vi "Configuration.vi"() -> ()   [LabVIEW 2017]
doc: "Demonstrates how to:\n- Discover SLSC devices\n- Reset SLSC devices\n- Rename SLSC devices\n- Add/remove SLSC chassis to/from the SLSC configuration file\n- Log in/out of an SLSC chassis, caching/deleting its login credentials\n- Update the firmware for an SLSC chassis\n- Open the web configuration page for an SLSC chassis"
uses:
  ConfigurationStates.ctl
  <vilib>/SLSC/Initialize Session without Resources.vi
  <vilib>/SLSC/Initialize Session with Devices.vi
  <vilib>/SLSC/Close Session.vi
  <vilib>/Platform/browser.llb/Open URL in Default Browser (string).vi
  <vilib>/SLSC/SLSC.lvlib
  <resource>/objmgr/slsc.rc
panel:
  in  "web config":bool
  in  "update firmware":bool
  out "device properties":string[][](table)
  in  "refresh":bool
  in  "logout":bool
  in  "login":bool
  in  "rename":bool
  in  "reset":bool
  in  "stop":bool
  in  "remove":bool
  in  "add":bool
  in  "devices":string(tree)="jasonSlsc-5"
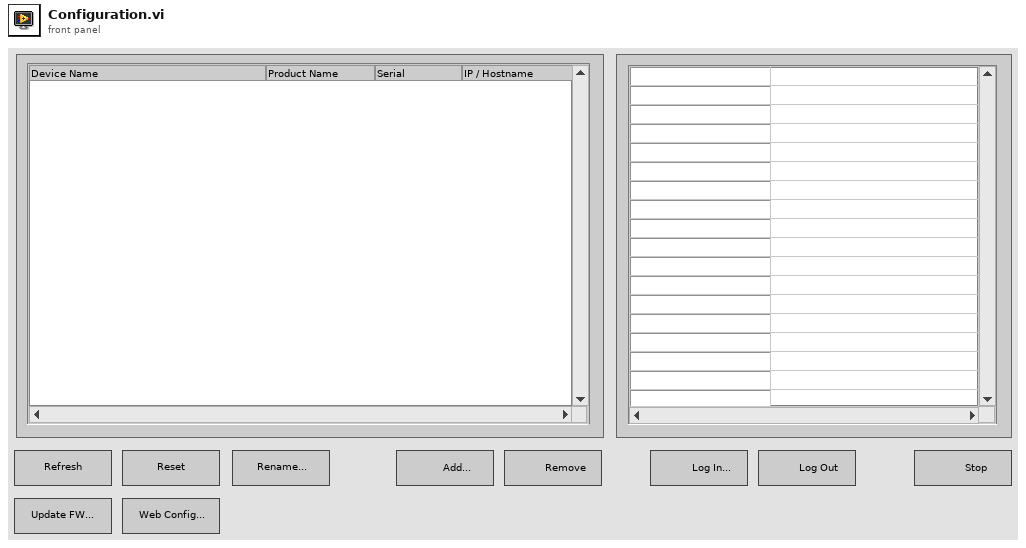
[diagram p1: front panel]
types:
  T1 = typedef "ConfigurationStates.ctl" = enum16{"Add", "Remove", "Rename", "Reset", "Login", "Logout", "Stop", "Refresh", "Update Firmware", "Web Config"}
  T2 = enum8{"Enabled", "Disabled", "Disabled and Grayed Out"}
  T3 = cluster{"hostname":string, "username":string, "password":string}
  T4 = cluster{"username":string, "password":string, "save credentials to disk":bool}
  T5 = cluster{"firmware path":path, "username":string, "password":string}
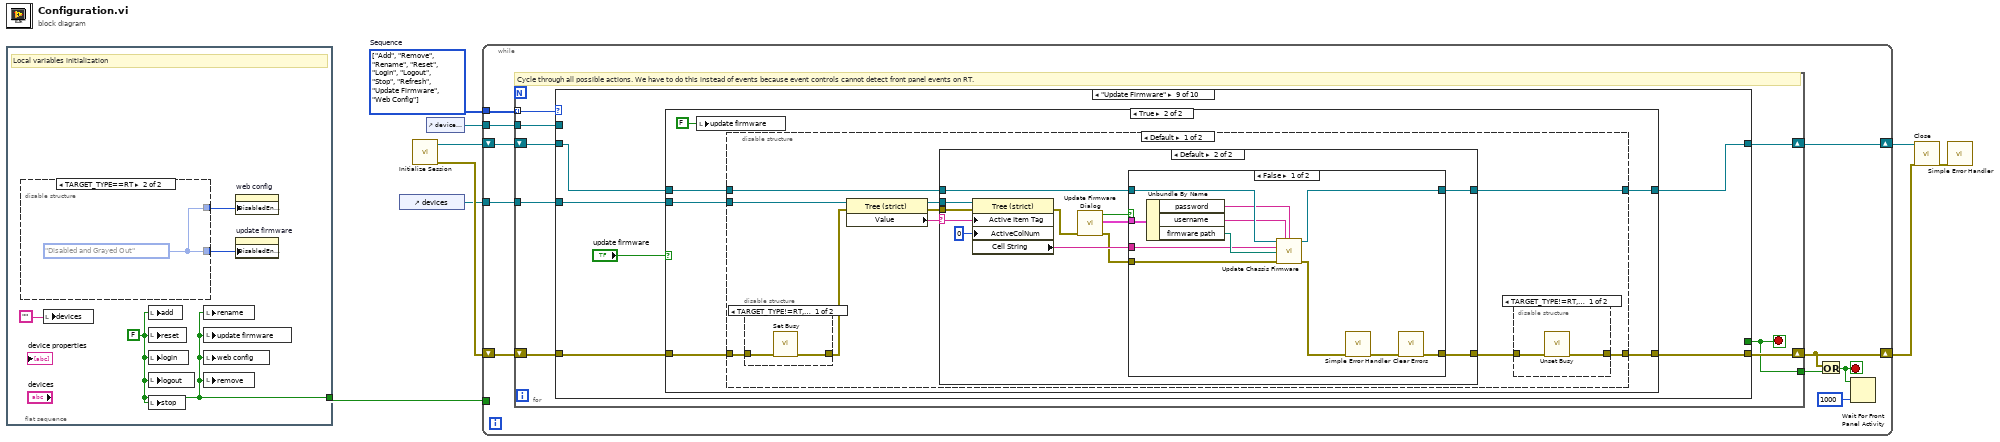
[diagram p0: block diagram]
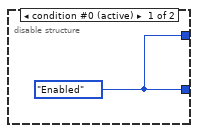
[diagram p2: hidden frame]
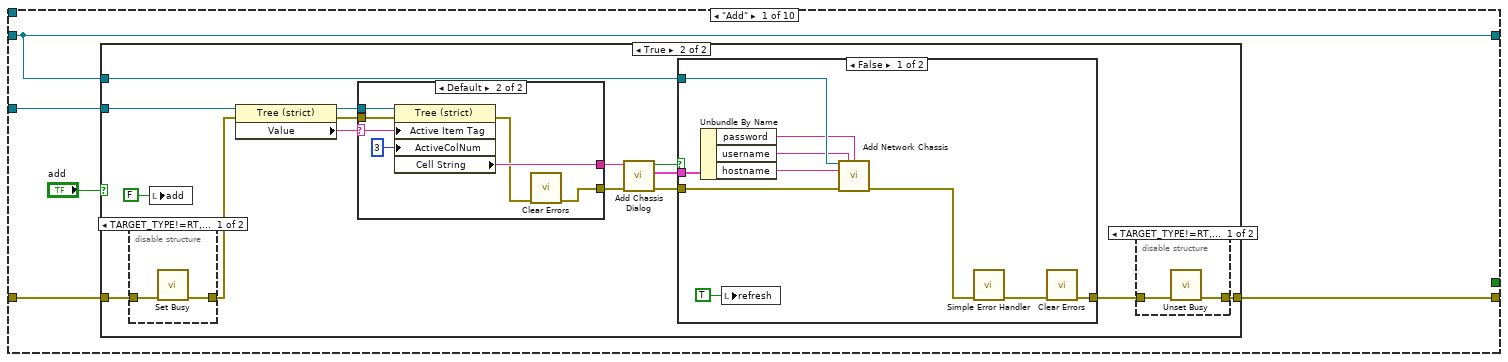
[diagram p3: hidden frame]
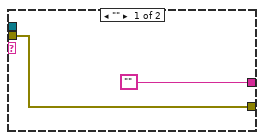
[diagram p5: hidden frame]
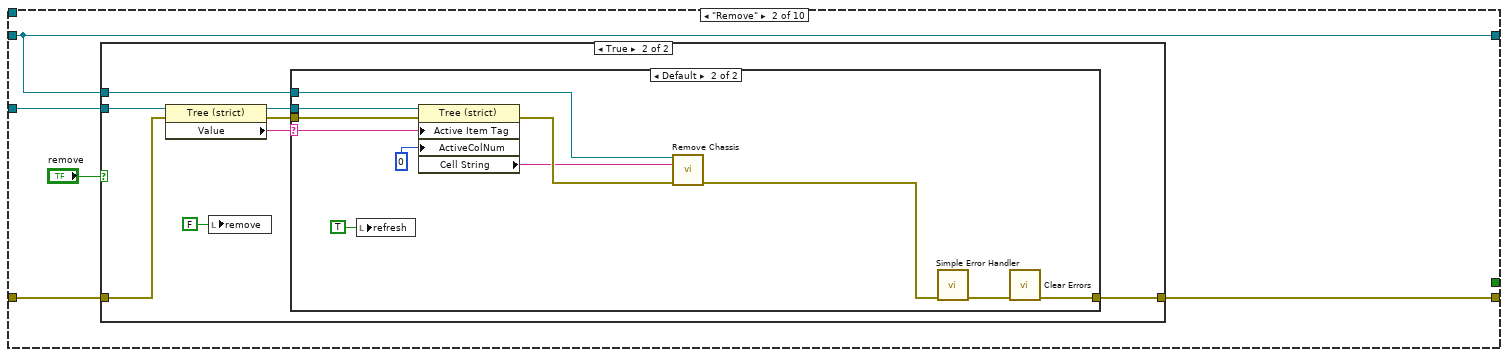
[diagram p9: hidden frame]
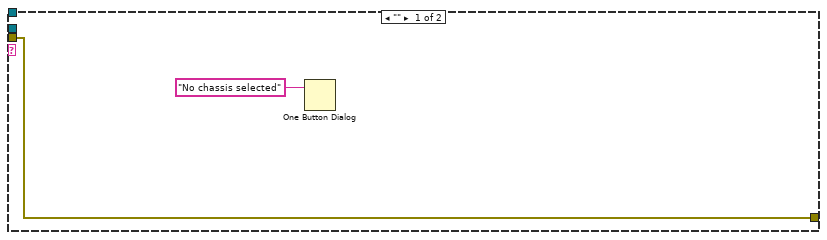
[diagram p11: hidden frame]
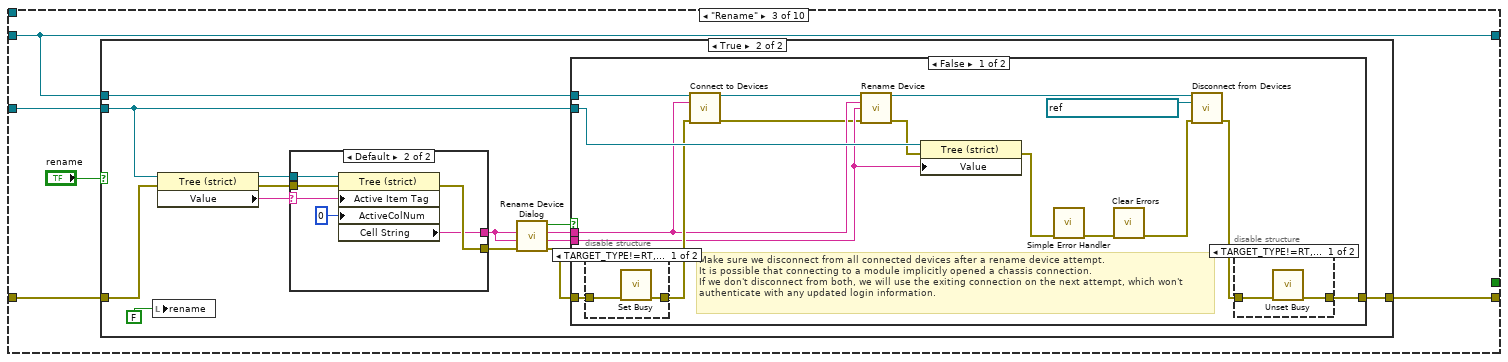
[diagram p12: hidden frame]
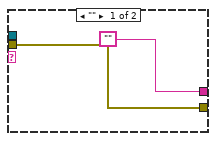
[diagram p14: hidden frame]
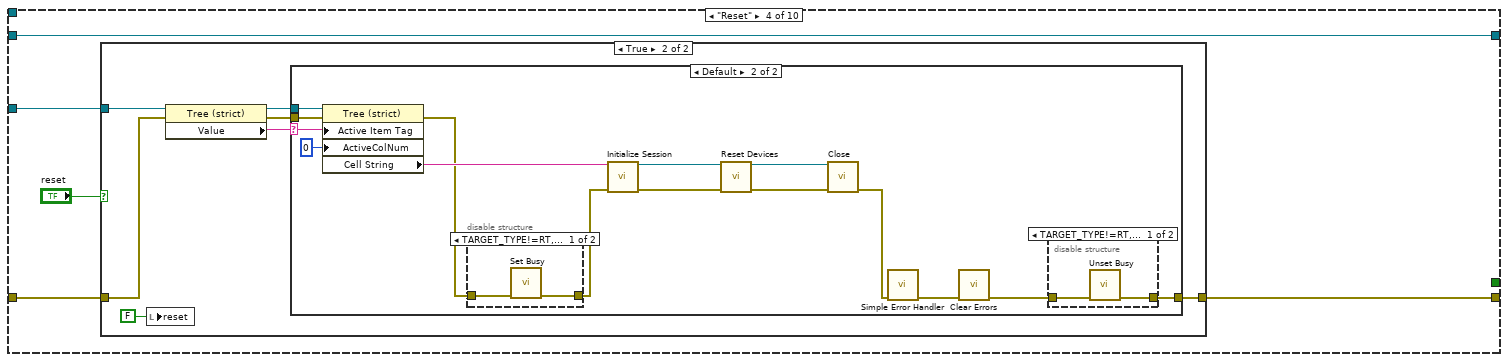
[diagram p18: hidden frame]
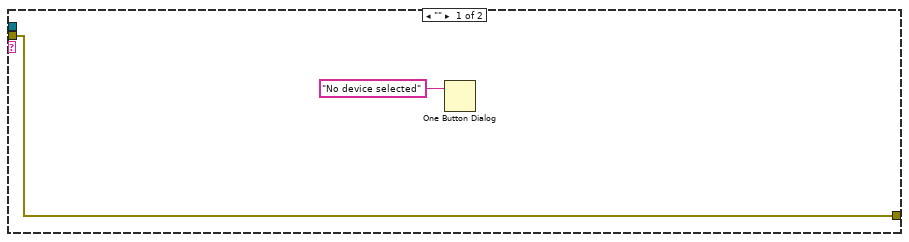
[diagram p20: hidden frame]
diagram:
  w4 = T1[] [enum."Add", enum."Remove", enum."Rename", enum."Reset", enum."Login", enum."Logout", enum."Stop", enum."Refresh", enum."Update Firmware", enum."Web Config"] items=["Add", "Remove", "Rename", "Reset", "Login", "Logout", "Stop", "Refresh", "Update Firmware", "Web Config"]  # Sequence
  n1 = flat-sequence {
    tunnel: [w13] -> w3
    frame #0 {
      w13 = FALSE
      # "Local variables initialization"
      n2 = disable-structure shown="TARGET_TYPE==RT" {
        disable-tunnel: [w14 w15] -> w12
        disable-tunnel: [w14 w15] -> w10
        frame condition #0 (active) {
          w14 = T2."Enabled" ("Disabled")
        }
        frame condition #1 {
          w15 = T2."Disabled and Grayed Out" ("Disabled")
        }
      }
      n3 = local write "devices"("") -> ()
      n4 = local write "add"(w13) -> ()
      n5 = local write "reset"(w13) -> ()
      n6 = local write "login"(w13) -> ()
      n7 = local write "logout"(w13) -> ()
      n8 = local write "stop"(w13) -> ()
      n9 = local write "rename"(w13) -> ()
      n10 = local write "update firmware"(w13) -> ()
      n11 = local write "web config"(w13) -> ()
      n12 = local write "remove"(w13) -> ()
      n13 = property on="web config" class="Bool (strict)"("DisabledEnum"=w10) -> ()  [unwired: 2 in, 2 out]
      n14 = property on="update firmware" class="Bool (strict)"("DisabledEnum"=w12) -> ()  [unwired: 2 in, 2 out]
    }
  }
  n15 = control-ref of="devices"() -> (w5:refnum<vi>)
  n16 = call-poly <vilib>:"Initialize Session.vi"() -> ("session out"=w6:refnum<k21>, "error out"=w9:errorcluster)  [unwired: 14 in]
  n17 = control-ref of="device properties"() -> (w1:refnum<vi>)
  n18 = while {
    shift-right: [w23] -> w8
    shift-left: w9 -> [w25]
    tunnel: w5 -> [w21]
    tunnel: w4 -> [w20]
    tunnel: w3 -> [_]
    shift-right: [w19] -> w2
    shift-left: w6 -> [w24]
    tunnel: w1 -> [w16]
    stop <- w17 stop-if-true
    n19 = for {
      tunnel: [w28] -> w22
      tunnel: w21 -> [w30]
      shift-right: [w31] -> w23
      shift-left: w25 -> [w33]
      tunnel: w20 -> [w29] mode=indexing
      shift-right: [w27] -> w19
      shift-left: w24 -> [w32]
      tunnel: w16 -> [w26]
      stop <- w28 stop-if-true
      # "Cycle through all possible actions. We have to do this instead of events because event controls cannot detect front panel events on RT."
      n20 = case shown="\"Update Firmware\"" w29 {
        tunnel: w33 -> [w37 w83 w111 w161 w198 w243 w268 w297 w368 w425]
        tunnel: w32 -> [w35 w81 w108 w159 w195 w240 w266 w289 w366 w427]
        tunnel: [w36 w82 w110 w160 w196 w241 w268 w274 w367 w424] -> w31
        tunnel: [_ _ _ _ _ _ "stop" _ _ _] -> w28
        tunnel: w30 -> [w34 w84 w112 w162 w197 w242 _ w291 w369 w428]
        tunnel: [w35 w81 w108 w159 w195 w240 w266 w294 w365 w426] -> w27
        tunnel: w26 -> [_ _ _ _ _ _ _ w292 _ _]
        frame "Add" {
          n21 = case shown="True" "add" {
            tunnel: w37 -> [w39 w53]
            tunnel: w35 -> [_ w52]
            tunnel: [w39 w51] -> w36
            tunnel: w34 -> [_ w40]
            frame False {
            }
            frame True {
              n22 = disable-structure shown="TARGET_TYPE!=RT, Default" {
                disable-tunnel: w53 -> [w68 w69]
                disable-tunnel: [w67 w69] -> w41
                frame condition #0 (active) {
                  n23 = call <vilib>:"Set Busy.vi"("error in (no error)"=w68) -> ("error out"=w67:errorcluster)  [unwired: 9 in, 1 out]
                }
                frame condition #1 {
                }
              }
              n24 = local write "add"(FALSE ("stop")) -> ()
              n25 = property class="Tree (strict)"(reference=w40, error in=w41) -> (reference out=w45:refnum<vi>, error out=w44:errorcluster, "Value"=w46:string)
              n26 = case shown="Default" w46 {
                selector: w46 -> [_ w59]
                tunnel: w44 -> [w56 w62]
                tunnel: w45 -> [_ w61]
                tunnel: [w56 w57] -> w42
                tunnel: ["" w60] -> w43
                frame "" {
                }
                frame Default {
                  n27 = property class="Tree (strict)"(reference=w61, error in=w62, "Active Item Tag"=w59, "ActiveColNum"=3 ("Active Cell:Active Column Number")) -> (error out=w58:errorcluster, "Cell String"=w60:string)  [unwired: 1 out]
                  n28 = call <vilib>:"Clear Errors.vi"("error in (no error)"=w58) -> ("error out"=w57:errorcluster)  [unwired: 5 in, 1 out]
                }
              }
              n29 = call "Add Chassis Dialog.vi"("error in (no error)"=w42, "hostname"=w43) -> ("error out"=w49:errorcluster, "Result"=w48:T3, "Cancelled?"=w50:bool)  [unwired: 7 in]
              n30 = case shown="False" w50 {
                tunnel: w52 -> [w79 _]
                tunnel: w48 -> [w78 _]
                tunnel: w49 -> [w76 w80]
                tunnel: [w73 w80] -> w54
                frame False {
                  n31 = Unbundle By Name(w78) -> ("password"=w71:string, "username"=w77:string, "hostname"=w70:string)
                  n32 = local write "refresh"(TRUE ("refresh")) -> ()
                  n33 = call <vilib>:"Add Network Chassis.vi"("session in"=w79, "username"=w77, "password"=w71, "chassis IP address/hostname"=w70, "error in (no error)"=w76) -> ("error out"=w75:errorcluster)  [unwired: 8 in, 2 out]
                  n34 = call <vilib>:"Simple Error Handler.vi"("error in (no error)"=w75) -> ("error out"=w74:errorcluster)  [unwired: 4 in, 4 out]
                  n35 = call <vilib>:"Clear Errors.vi"("error in (no error)"=w74) -> ("error out"=w73:errorcluster)  [unwired: 5 in, 1 out]
                }
                frame True {
                }
              }
              n36 = disable-structure shown="TARGET_TYPE!=RT, Default" {
                disable-tunnel: w54 -> [w65 w66]
                disable-tunnel: [w64 w66] -> w51
                frame condition #0 (active) {
                  n37 = call <vilib>:"Unset Busy.vi"("error in (no error)"=w65) -> ("error out"=w64:errorcluster)  [unwired: 10 in]
                }
                frame condition #1 {
                }
              }
            }
          }
        }
        frame "Remove" {
          n38 = case shown="True" "remove" {
            tunnel: w81 -> [_ w91]
            tunnel: w84 -> [_ w90]
            tunnel: w83 -> [w86 w89]
            tunnel: [w86 w88] -> w82
            frame False {
            }
            frame True {
              n39 = property class="Tree (strict)"(reference=w90, error in=w89) -> (reference out=w93:refnum<vi>, error out=w92:errorcluster, "Value"=w94:string)
              n40 = local write "remove"(FALSE ("stop")) -> ()
              n41 = case shown="Default" w94 {
                selector: w94 -> [_ w98]
                tunnel: w92 -> [w96 w106]
                tunnel: w93 -> [_ w105]
                tunnel: w91 -> [_ w104]
                tunnel: [w96 w102] -> w88
                frame "" {
                  n42 = One Button Dialog(message="No chassis selected") -> ()  [unwired: 1 in, 1 out]
                }
                frame Default {
                  n43 = local write "refresh"(TRUE ("refresh")) -> ()
                  n44 = property class="Tree (strict)"(reference=w105, error in=w106, "Active Item Tag"=w98, "ActiveColNum"=0 ("Active Cell:Active Column Number")) -> (error out=w103:errorcluster, "Cell String"=w99:string)  [unwired: 1 out]
                  n45 = call <vilib>:"Remove Chassis.vi"("session in"=w104, "chassis"=w99, "error in (no error)"=w103) -> ("error out"=w101:errorcluster)  [unwired: 11 in, 1 out]
                  n46 = call <vilib>:"Simple Error Handler.vi"("error in (no error)"=w101) -> ("error out"=w100:errorcluster)  [unwired: 4 in, 4 out]
                  n47 = call <vilib>:"Clear Errors.vi"("error in (no error)"=w100) -> ("error out"=w102:errorcluster)  [unwired: 5 in, 1 out]
                }
              }
            }
          }
        }
        frame "Rename" {
          n48 = case shown="True" "rename" {
            tunnel: w112 -> [_ w115]
            tunnel: w111 -> [w113 w117]
            tunnel: [w113 w119] -> w110
            tunnel: w108 -> [_ w114]
            frame False {
            }
            frame True {
              n49 = local write "rename"(FALSE ("stop")) -> ()
              n50 = property class="Tree (strict)"(reference=w115, error in=w117) -> (reference out=w126:refnum<vi>, error out=w125:errorcluster, "Value"=w127:string)
              n51 = case shown="Default" w127 {
                selector: w127 -> [_ w130]
                tunnel: w125 -> [w129 w134]
                tunnel: w126 -> [_ w133]
                tunnel: [w129 w132] -> w116
                tunnel: ["" w131] -> w120
                frame "" {
                }
                frame Default {
                  n52 = property class="Tree (strict)"(reference=w133, error in=w134, "Active Item Tag"=w130, "ActiveColNum"=0 ("Active Cell:Active Column Number")) -> (error out=w132:errorcluster, "Cell String"=w131:string)  [unwired: 1 out]
                }
              }
              n53 = call "Rename Device Dialog.vi"("error in (no error)"=w116, "new device name"=w120, "old device name"=w120) -> ("error out"=w118:errorcluster, "new device name out"=w122:string, "old device name out"=w123:string, "Cancelled?"=w124:bool)  [unwired: 5 in]
              n54 = case shown="False" w124 {
                tunnel: w123 -> [w145 _]
                tunnel: w122 -> [w144 _]
                tunnel: w118 -> [w149 w158]
                tunnel: [w150 w158] -> w119
                tunnel: w115 -> [w148 _]
                tunnel: w114 -> [w146 _]
                frame False {
                  # "Make sure we disconnect from all connected devices after a rename device attempt.\nIt is possible that connecting to a module implicitly opened a chassis connection.\nIf we don't disconnect from both, we will use the exiting connection on the next attempt, which won't authenticate with any updated login information."
                  n55 = disable-structure shown="TARGET_TYPE!=RT, Default" {
                    disable-tunnel: w149 -> [w152 w154]
                    disable-tunnel: [w153 w154] -> w147
                    frame condition #0 (active) {
                      n56 = call <vilib>:"Set Busy.vi"("error in (no error)"=w152) -> ("error out"=w153:errorcluster)  [unwired: 9 in, 1 out]
                    }
                    frame condition #1 {
                    }
                  }
                  n57 = call <vilib>:"Connect to Devices.vi"("session in"=w146, "devices"=w145, "error in (no error)"=w147) -> ("session out"=w142:refnum<k21>, "error out"=w141:errorcluster)  [unwired: 11 in]
                  n58 = call <vilib>:"Rename Device.vi"("session in"=w142, "device"=w145, "new device name"=w144, "error in (no error)"=w141) -> ("session out"=w138:refnum<k21>, "error out"=w140:errorcluster)  [unwired: 10 in]
                  n59 = property class="Tree (strict)"(reference=w148, error in=w140, "Value"=w144) -> (error out=w143:errorcluster)  [unwired: 1 out]
                  n60 = call <vilib>:"Simple Error Handler.vi"("error in (no error)"=w143) -> ("error out"=w151:errorcluster)  [unwired: 4 in, 4 out]
                  n61 = call <vilib>:"Clear Errors.vi"("error in (no error)"=w151) -> ("error out"=w136:errorcluster)  [unwired: 5 in, 1 out]
                  n62 = call <vilib>:"Disconnect from Devices.vi"("session in"=w138, "devices"=refnum<k21> "$ConnectedDevices", "error in (no error)"=w136) -> ("error out"=w139:errorcluster)  [unwired: 11 in, 1 out]
                  n63 = disable-structure shown="TARGET_TYPE!=RT, Default" {
                    disable-tunnel: w139 -> [w156 w157]
                    disable-tunnel: [w155 w157] -> w150
                    frame condition #0 (active) {
                      n64 = call <vilib>:"Unset Busy.vi"("error in (no error)"=w156) -> ("error out"=w155:errorcluster)  [unwired: 10 in]
                    }
                    frame condition #1 {
                    }
                  }
                }
                frame True {
                }
              }
            }
          }
        }
        frame "Reset" {
          n65 = case shown="True" "reset" {
            tunnel: w162 -> [_ w169]
            tunnel: w161 -> [w164 w168]
            tunnel: [w164 w165] -> w160
            frame False {
            }
            frame True {
              n66 = local write "reset"(FALSE ("stop")) -> ()
              n67 = property class="Tree (strict)"(reference=w169, error in=w168) -> (reference out=w170:refnum<vi>, error out=w166:errorcluster, "Value"=w171:string)
              n68 = case shown="Default" w171 {
                selector: w171 -> [_ w184]
                tunnel: w166 -> [w173 w187]
                tunnel: w170 -> [_ w186]
                tunnel: [w173 w174] -> w165
                frame "" {
                  n69 = One Button Dialog(message="No device selected") -> ()  [unwired: 1 in, 1 out]
                }
                frame Default {
                  n70 = property class="Tree (strict)"(reference=w186, error in=w187, "Active Item Tag"=w184, "ActiveColNum"=0 ("Active Cell:Active Column Number")) -> (error out=w177:errorcluster, "Cell String"=w181:string)  [unwired: 1 out]
                  n71 = disable-structure shown="TARGET_TYPE!=RT, Default" {
                    disable-tunnel: w177 -> [w193 w194]
                    disable-tunnel: [w192 w194] -> w176
                    frame condition #0 (active) {
                      n72 = call <vilib>:"Set Busy.vi"("error in (no error)"=w193) -> ("error out"=w192:errorcluster)  [unwired: 9 in, 1 out]
                    }
                    frame condition #1 {
                    }
                  }
                  n73 = call-poly <vilib>:"Initialize Session.vi"("devices"=w181, "error in (no error)"=w176) -> ("session out"=w183:refnum<k21>, "error out"=w182:errorcluster)  [unwired: 12 in]
                  n74 = call <vilib>:"Reset Devices.vi"("session in"=w183, "error in (no error)"=w182) -> ("session out"=w178:refnum<k21>, "error out"=w180:errorcluster)  [unwired: 12 in]
                  n75 = call-poly <vilib>:"Close.vi"("session in"=w178, "error in (no error)"=w180) -> ("error out"=w179:errorcluster)  [unwired: 13 in]
                  n76 = call <vilib>:"Simple Error Handler.vi"("error in (no error)"=w179) -> ("error out"=w185:errorcluster)  [unwired: 4 in, 4 out]
                  n77 = call <vilib>:"Clear Errors.vi"("error in (no error)"=w185) -> ("error out"=w175:errorcluster)  [unwired: 5 in, 1 out]
                  n78 = disable-structure shown="TARGET_TYPE!=RT, Default" {
                    disable-tunnel: w175 -> [w190 w191]
                    disable-tunnel: [w189 w191] -> w174
                    frame condition #0 (active) {
                      n79 = call <vilib>:"Unset Busy.vi"("error in (no error)"=w190) -> ("error out"=w189:errorcluster)  [unwired: 10 in]
                    }
                    frame condition #1 {
                    }
                  }
                }
              }
            }
          }
        }
        frame "Login" {
          n80 = case shown="True" "login" {
            tunnel: w195 -> [_ w205]
            tunnel: w198 -> [w200 w204]
            tunnel: w197 -> [_ w203]
            tunnel: [w200 w202] -> w196
            frame False {
            }
            frame True {
              n81 = local write "login"(FALSE ("stop")) -> ()
              n82 = property class="Tree (strict)"(reference=w203, error in=w204) -> (reference out=w207:refnum<vi>, error out=w206:errorcluster, "Value"=w208:string)
              n83 = case shown="Default" w208 {
                selector: w208 -> [_ w219]
                tunnel: w206 -> [w209 w221]
                tunnel: w207 -> [_ w220]
                tunnel: [w209 w214] -> w202
                tunnel: w205 -> [_ w217]
                frame "" {
                }
                frame Default {
                  n84 = property class="Tree (strict)"(reference=w220, error in=w221, "Active Item Tag"=w219, "ActiveColNum"=0 ("Active Cell:Active Column Number")) -> (error out=w216:errorcluster, "Cell String"=w218:string)  [unwired: 1 out]
                  n85 = disable-structure shown="TARGET_TYPE!=RT, Default" {
                    disable-tunnel: w216 -> [w227 w228]
                    disable-tunnel: [w226 w228] -> w211
                    frame condition #0 (active) {
                      n86 = call <vilib>:"Set Busy.vi"("error in (no error)"=w227) -> ("error out"=w226:errorcluster)  [unwired: 9 in, 1 out]
                    }
                    frame condition #1 {
                    }
                  }
                  n87 = call "Log In Dialog.vi"("error in (no error)"=w211) -> ("error out"=w210:errorcluster, "Result"=w212:T4, "Cancelled?"=w213:bool)  [unwired: 8 in]
                  n88 = case shown="False" w213 {
                    tunnel: w212 -> [w238 _]
                    tunnel: w210 -> [w237 w239]
                    tunnel: [w234 w239] -> w215
                    tunnel: w218 -> [w233 _]
                    tunnel: w217 -> [w232 _]
                    frame False {
                      n89 = Unbundle By Name(w238) -> ("password"=w229:string, "username"=w231:string, "save credentials to disk"=w230:bool)
                      n90 = call <vilib>:"Log In.vi"("session in"=w232, "username"=w231, "password"=w229, "chassis"=w233, "error in (no error)"=w237, "save credentials to disk? (F)"=w230) -> ("error out"=w236:errorcluster)  [unwired: 8 in, 1 out]
                      n91 = call <vilib>:"Simple Error Handler.vi"("error in (no error)"=w236) -> ("error out"=w235:errorcluster)  [unwired: 4 in, 4 out]
                      n92 = call <vilib>:"Clear Errors.vi"("error in (no error)"=w235) -> ("error out"=w234:errorcluster)  [unwired: 5 in, 1 out]
                    }
                    frame True {
                    }
                  }
                  n93 = disable-structure shown="TARGET_TYPE!=RT, Default" {
                    disable-tunnel: w215 -> [w224 w225]
                    disable-tunnel: [w223 w225] -> w214
                    frame condition #0 (active) {
                      n94 = call <vilib>:"Unset Busy.vi"("error in (no error)"=w224) -> ("error out"=w223:errorcluster)  [unwired: 10 in]
                    }
                    frame condition #1 {
                    }
                  }
                }
              }
            }
          }
        }
        frame "Logout" {
          n95 = case shown="True" "logout" {
            tunnel: w240 -> [_ w250]
            tunnel: w243 -> [w245 w249]
            tunnel: w242 -> [_ w248]
            tunnel: [w245 w247] -> w241
            frame False {
            }
            frame True {
              n96 = property class="Tree (strict)"(reference=w248, error in=w249) -> (reference out=w252:refnum<vi>, error out=w251:errorcluster, "Value"=w253:string)
              n97 = local write "logout"(FALSE ("stop")) -> ()
              n98 = case shown="Default" w253 {
                selector: w253 -> [_ w256]
                tunnel: w251 -> [w255 w264]
                tunnel: w252 -> [_ w263]
                tunnel: w250 -> [_ w262]
                tunnel: [w255 w260] -> w247
                frame "" {
                  n99 = One Button Dialog(message="No chassis selected") -> ()  [unwired: 1 in, 1 out]
                }
                frame Default {
                  n100 = property class="Tree (strict)"(reference=w263, error in=w264, "Active Item Tag"=w256, "ActiveColNum"=0 ("Active Cell:Active Column Number")) -> (error out=w261:errorcluster, "Cell String"=w257:string)  [unwired: 1 out]
                  n101 = call <vilib>:"Log Out.vi"("session in"=w262, "chassis"=w257, "error in (no error)"=w261) -> ("error out"=w259:errorcluster)  [unwired: 11 in, 1 out]
                  n102 = call <vilib>:"Simple Error Handler.vi"("error in (no error)"=w259) -> ("error out"=w258:errorcluster)  [unwired: 4 in, 4 out]
                  n103 = call <vilib>:"Clear Errors.vi"("error in (no error)"=w258) -> ("error out"=w260:errorcluster)  [unwired: 5 in, 1 out]
                }
              }
            }
          }
        }
        frame "Stop" {
          n104 = case shown="True" "stop" {
            frame False {
            }
            frame True {
              n105 = local write "stop"(FALSE ("stop")) -> ()
            }
          }
        }
        frame "Refresh" {
          n106 = disable-structure shown="TARGET_TYPE!=RT, Default" {
            disable-tunnel: w297 -> [w359 w363]
            disable-tunnel: [w358 w363] -> w271
            disable-tunnel: [w357 _] -> w298
            frame condition #0 (active) {
              n107 = property class="VI"(error in=w359) -> (error out=w361:errorcluster, "Panel"=w362:refnum<vi>)  [unwired: 1 in, 1 out]
              n108 = property class="Pnl"(reference=w362, error in=w361, "DeferPanUpdts"=TRUE ("Defer Panel Updates")) -> (reference out=w357:refnum<vi>, error out=w358:errorcluster)
            }
            frame condition #1 {
            }
          }
          n109 = case shown="True" "refresh" {
            tunnel: [w344 w346] -> w270
            tunnel: w271 -> [w344 w345]
            frame False {
            }
            frame True {
              n110 = local write "refresh"(FALSE ("refresh")) -> ()
              n111 = invoke on="devices" class="Tree (strict)" method="Edit Tree Items.Delete"("tag"="", "Delete Children"=TRUE ("refresh")) -> (error out=w347:errorcluster)  [unwired: 3 in, 4 out]
              n112 = Merge Errors(w347, w345) -> (w346:errorcluster)
            }
          }
          n113 = property class="SLSC Session"(reference=w289, error in=w270) -> (reference out=w288:refnum<k21>, error out=w287:errorcluster, "Sys.ConfigChangeCount"=w284:u64)
          n114 = feedback #1(u64 0 ("Sys.ConfigChangeCount")) -> (w285:u64)
          n115 = feedback-in #1(w284) -> ()
          n116 = Not Equal?(x=w284, y=w285) -> (x != y?=w282:bool)
          n117 = Or(x=w282, y="refresh") -> (x .or. y?=w283:bool)
          n118 = case shown="True" w283 {
            tunnel: [w307 w315] -> w296
            tunnel: [w309 w314] -> w295
            tunnel: w291 -> [w308 w313]
            tunnel: [w308 w312] -> w290
            tunnel: w288 -> [w309 w311]
            tunnel: w287 -> [w307 w310]
            frame False {
            }
            frame True {
              n119 = call "Update Config Tree.vi"("error in (no error)"=w310, "devices"=w313, "session in"=w311) -> ("error out"=w315:errorcluster, "devices out"=w312:refnum<vi>, "session out"=w314:refnum<k21>)  [unwired: 6 in]
            }
          }
          n120 = property class="Tree (strict)"(reference=w290, error in=w296) -> (reference out=w278:refnum<vi>, error out=w277:errorcluster, "Value"=w273:string, "All Tags"=w280:string[])
          n121 = Search 1D Array(1D array=w280, element=w273) -> (index of element=w279:i32)  [unwired: 1 in]
          n122 = case shown="-1" w279 {
            tunnel: w278 -> [w300 w305]
            tunnel: w277 -> [w301 w306]
            tunnel: [w300 w304] -> w276
            tunnel: [w301 w303] -> w275
            tunnel: w273 -> [w299 _]
            tunnel: [w299 w302] -> w272
            frame Default {
              # "Tag is valid"
            }
            frame -1 {
              w302 = ""
              # "Tag is no longer valid. Clear control value to avoid accessing invalid tree items."
              n123 = property class="Tree (strict)"(reference=w305, error in=w306, "Value"=w302) -> (reference out=w304:refnum<vi>, error out=w303:errorcluster)
            }
          }
          n124 = case shown="Default" w272 {
            selector: w272 -> [_ w335]
            tunnel: w295 -> [w319 w334]
            tunnel: [w319 w328] -> w294
            tunnel: w275 -> [w320 w330]
            tunnel: w276 -> [_ w333]
            tunnel: [w321 w329] -> w293
            tunnel: "refresh" -> [_ w332]
            tunnel: w292 -> [w316 w331]
            frame "" {
              n125 = property class="Tbl (strict)"(reference=w316, error in=w320, "Row Headers[]"=string[] [] ("Row Header Strings[]"), "Value"=string[][] []) -> (error out=w321:errorcluster)  [unwired: 1 out]
            }
            frame Default {
              n126 = property class="Tree (strict)"(reference=w333, error in=w330, "Active Item Tag"=w335, "ActiveColNum"=0 ("Active Cell:Active Column Number")) -> (error out=w326:errorcluster, "Cell String"=w323:string)  [unwired: 1 out]
              n127 = feedback #2() -> (w322:string)  [unwired: 1 in]
              n128 = feedback-in #2(w323) -> ()
              n129 = Not Equal?(x=w323, y=w322) -> (x != y?=w325:bool)
              n130 = Or(x=w325, y=w332) -> (x .or. y?=w324:bool)
              n131 = case shown="True" w324 {
                tunnel: w323 -> [_ w343]
                tunnel: w326 -> [w336 w342]
                tunnel: w334 -> [w337 w341]
                tunnel: [w337 w340] -> w328
                tunnel: [w336 w339] -> w329
                tunnel: w331 -> [_ w338]
                frame False {
                }
                frame True {
                  n132 = call "Update Device Properties Table.vi"("session in"=w341, "device"=w343, "device properties"=w338, "error in (no error)"=w342) -> ("session out"=w340:refnum<k21>, "error out"=w339:errorcluster)  [unwired: 10 in]
                }
              }
            }
          }
          n133 = disable-structure shown="TARGET_TYPE!=RT, Default" {
            disable-tunnel: w298 -> [w355 _]
            disable-tunnel: w293 -> [w352 w356]
            disable-tunnel: [w351 w356] -> w274
            frame condition #0 (active) {
              n134 = property class="Pnl"(reference=w355, "DeferPanUpdts"=FALSE ("Defer Panel Updates")) -> (error out=w353:errorcluster)  [unwired: 1 in, 1 out]
              n135 = Merge Errors(w352, w353) -> (w351:errorcluster)
            }
            frame condition #1 {
            }
          }
        }
        frame "Update Firmware" {
          n136 = case shown="True" "update firmware" {
            tunnel: w369 -> [_ w377]
            tunnel: w368 -> [w371 w375]
            tunnel: [w371 w374] -> w367
            tunnel: w366 -> [w370 w373]
            tunnel: [w370 w372] -> w365
            frame False {
            }
            frame True {
              n137 = local write "update firmware"(FALSE ("update firmware")) -> ()
              n138 = disable-structure shown="Default" {
                disable-tunnel: w377 -> [w384 _]
                disable-tunnel: w375 -> [w383 w421]
                disable-tunnel: [w380 w421] -> w374
                disable-tunnel: w373 -> [w379 w422]
                disable-tunnel: [w378 w422] -> w372
                frame condition #0 (active) {
                  n139 = disable-structure shown="TARGET_TYPE!=RT, Default" {
                    disable-tunnel: w383 -> [w392 w393]
                    disable-tunnel: [w391 w393] -> w382
                    frame condition #0 (active) {
                      n140 = call <vilib>:"Set Busy.vi"("error in (no error)"=w392) -> ("error out"=w391:errorcluster)  [unwired: 9 in, 1 out]
                    }
                    frame condition #1 {
                    }
                  }
                  n141 = property class="Tree (strict)"(reference=w384, error in=w382) -> (reference out=w386:refnum<vi>, error out=w385:errorcluster, "Value"=w387:string)
                  n142 = case shown="Default" w387 {
                    selector: w387 -> [_ w404]
                    tunnel: w385 -> [w395 w406]
                    tunnel: w386 -> [_ w405]
                    tunnel: [w395 w398] -> w381
                    tunnel: w379 -> [w394 w397]
                    tunnel: [w394 w396] -> w378
                    frame "" {
                    }
                    frame Default {
                      n143 = property class="Tree (strict)"(reference=w405, error in=w406, "Active Item Tag"=w404, "ActiveColNum"=0 ("Active Cell:Active Column Number")) -> (error out=w403:errorcluster, "Cell String"=w400:string)  [unwired: 1 out]
                      n144 = call "Update Firmware Dialog.vi"("error in (no error)"=w403) -> ("error out"=w399:errorcluster, "Result"=w401:T5, "Cancelled?"=w402:bool)  [unwired: 8 in]
                      n145 = case shown="False" w402 {
                        tunnel: w401 -> [w418 _]
                        tunnel: w400 -> [w408 _]
                        tunnel: w399 -> [w411 w420]
                        tunnel: [w416 w420] -> w398
                        tunnel: w397 -> [w415 w419]
                        tunnel: [w409 w419] -> w396
                        frame False {
                          n146 = Unbundle By Name(w418) -> ("password"=w413:string, "username"=w414:string, "firmware path"=w412:path)
                          n147 = call <vilib>:"Update Chassis Firmware.vi"("session in"=w415, "username"=w414, "password"=w413, "chassis"=w408, "firmware path"=w412, "error in (no error)"=w411) -> ("session out"=w409:refnum<k21>, "error out"=w410:errorcluster)  [unwired: 8 in]
                          n148 = call <vilib>:"Simple Error Handler.vi"("error in (no error)"=w410) -> ("error out"=w417:errorcluster)  [unwired: 4 in, 4 out]
                          n149 = call <vilib>:"Clear Errors.vi"("error in (no error)"=w417) -> ("error out"=w416:errorcluster)  [unwired: 5 in, 1 out]
                        }
                        frame True {
                        }
                      }
                    }
                  }
                  n150 = disable-structure shown="TARGET_TYPE!=RT, Default" {
                    disable-tunnel: w381 -> [w389 w390]
                    disable-tunnel: [w388 w390] -> w380
                    frame condition #0 (active) {
                      n151 = call <vilib>:"Unset Busy.vi"("error in (no error)"=w389) -> ("error out"=w388:errorcluster)  [unwired: 10 in]
                    }
                    frame condition #1 {
                    }
                  }
                }
                frame condition #1 {
                  n152 = One Button Dialog(message="Firmware update is not supported on this platform.") -> ()  [unwired: 1 in, 1 out]
                }
              }
            }
          }
        }
        frame "Web Config" {
          n153 = case shown="True" "web config" {
            tunnel: w427 -> [w430 w435]
            tunnel: w428 -> [_ w436]
            tunnel: [w430 w434] -> w426
            tunnel: w425 -> [w431 w433]
            tunnel: [w431 w432] -> w424
            frame False {
            }
            frame True {
              n154 = local write "web config"(FALSE ("web config")) -> ()
              n155 = disable-structure shown="Default" {
                disable-tunnel: w436 -> [w445 _]
                disable-tunnel: w435 -> [w442 _]
                disable-tunnel: [w441 _] -> w434
                disable-tunnel: w433 -> [w440 _]
                disable-tunnel: [w439 _] -> w432
                frame condition #0 (active) {
                  n156 = property class="Tree (strict)"(reference=w445, error in=w440) -> (reference out=w438:refnum<vi>, error out=w443:errorcluster, "Value"=w444:string)
                  n157 = case shown="Default" w444 {
                    selector: w444 -> [_ w451]
                    tunnel: w443 -> [w446 w461]
                    tunnel: w442 -> [w447 w459]
                    tunnel: [w447 w458] -> w441
                    tunnel: [w446 w448] -> w439
                    tunnel: w438 -> [_ w452]
                    frame "" {
                    }
                    frame Default {
                      n158 = property class="Tree (strict)"(reference=w452, error in=w461, "Active Item Tag"=w451, "ActiveColNum"=0 ("Active Cell:Active Column Number")) -> (error out=w457:errorcluster, "Cell String"=w460:string)  [unwired: 1 out]
                      n159 = call <vilib>:"Get Chassis IP or Hostname.vi"("session in"=w459, "chassis"=w460, "error in (no error)"=w457) -> ("session out"=w458:refnum<k21>, "chassis IP address/hostname"=w455:string, "error out"=w453:errorcluster)  [unwired: 10 in]
                      n160 = Concatenate Strings("http://", w455) -> (w454:string)
                      n161 = call-poly <vilib>:"Open URL in Default Browser.vi"("error in (no error)"=w453, "URL"=w454) -> ("error out"=w449:errorcluster)  [unwired: 4 in, 1 out]
                      n162 = call <vilib>:"Simple Error Handler.vi"("error in (no error)"=w449) -> ("error out"=w450:errorcluster)  [unwired: 4 in, 4 out]
                      n163 = call <vilib>:"Clear Errors.vi"("error in (no error)"=w450) -> ("error out"=w448:errorcluster)  [unwired: 5 in, 1 out]
                    }
                  }
                }
                frame condition #1 {
                  n164 = One Button Dialog(message="Opening a web browser is not supported on this platform.") -> ()  [unwired: 1 in, 1 out]
                }
              }
            }
          }
        }
      }
    }
    n165 = Or(x=w23, y=w22) -> (x .or. y?=w17:bool)
    n166 = Wait For Front Panel Activity(1:1000 ("timeout ms (-1 never timeout)"), 3:w17) -> ()  [unwired: 1 in, 1 out]
  }
  n167 = call-poly <vilib>:"Close.vi"("session in"=w2, "error in (no error)"=w8) -> ("error out"=w7:errorcluster)  [unwired: 13 in]
  n168 = call <vilib>:"Simple Error Handler.vi"("error in (no error)"=w7) -> ()  [unwired: 4 in, 5 out]
